vi "Autonomous Independent.vi"   [LabVIEW 2013]
doc: "This VI is called when autonomous begins, and will automatically be terminated when autonomous ends. You can carry out timed or sensor driven robot movement independently without needing to return to the caller."
uses:
  Robot Global Data.vi
  <vilib>/Rock Robotics/WPI/RobotDrive/WPI_RobotDriveGetSetRefNum.vi
panel:
  # "Be sure to right-click and choose Data Operations>>Make Current Value default if you want to save the array values with the VI"
types:
  T1 = enum16{"ToPos2", "ToPos1", "Fire", "Wait", "ESTOP", "Reset", "ToLowPower", "ToHighPower"}
  T2 = typedef "WPI_MotorControlDeviceRef.ctl" = cluster{"DeviceStatus":errorcluster, "Type":enum16{"PWM", "CAN"}, "PWM":cluster{"Digital Module":T3, "PWM Channel":T4, "DeadBand":T5}, "CAN":cluster{"Device Number":u8, "Control Mode":T6, "Semaphore":T7, "Max Vout":dbl}, "Invert":bool, "TransformRef":T8, "InvTransformRef":T8}
  T3 = typedef "FPGA_TypedefDigitalModule.ctl" = enum16{"Digital Module 1", "Digital Module 2"}
  T4 = typedef "FPGA_DIOPWMChannel.ctl" = enum8{"PWM 1", "PWM 2", "PWM 3", "PWM 4", "PWM 5", "PWM 6", "PWM 7", "PWM 8", "PWM 9", "PWM 10", "Invalid"}
  T5 = typedef "WPI_PWMDeadband.ctl" = cluster{"Name":string, "maxPositivePwm":i32, "minPositivePwm":i32, "centerPwm":i32, "maxNegativePwm":i32, "minNegativePwm":i32, "angularRange":u16}
  T6 = typedef "WPI_CANJaguar_ControlMode.ctl" = enum8{"Percent VBus", "Current", "Speed", "Position", "Voltage"}
  T7 = typedef "Semaphore RefNum" = refnum<k1>
  T8 = typedef "WPI_PWMTransform_ConPane.ctl" = refnum<vi>
  T9 = cluster{"UpLimit":bool, "Up2":bool, "Center":bool, "Down2":bool, "DownLimit":bool, "HighPowerLimit":bool, "EncoderRRate":dbl, "EncoderLRate":dbl, "ThumperE":dbl, "EncoderRDis":dbl, "EncoderLDis":dbl}
  T10 = typedef "WPI_RobotDriveDevRef.ctl" = cluster{"DevStatus":errorcluster, "Motors[]":T2[], "Square Inputs":bool, "Max Output":dbl, "Isochronous":bool}
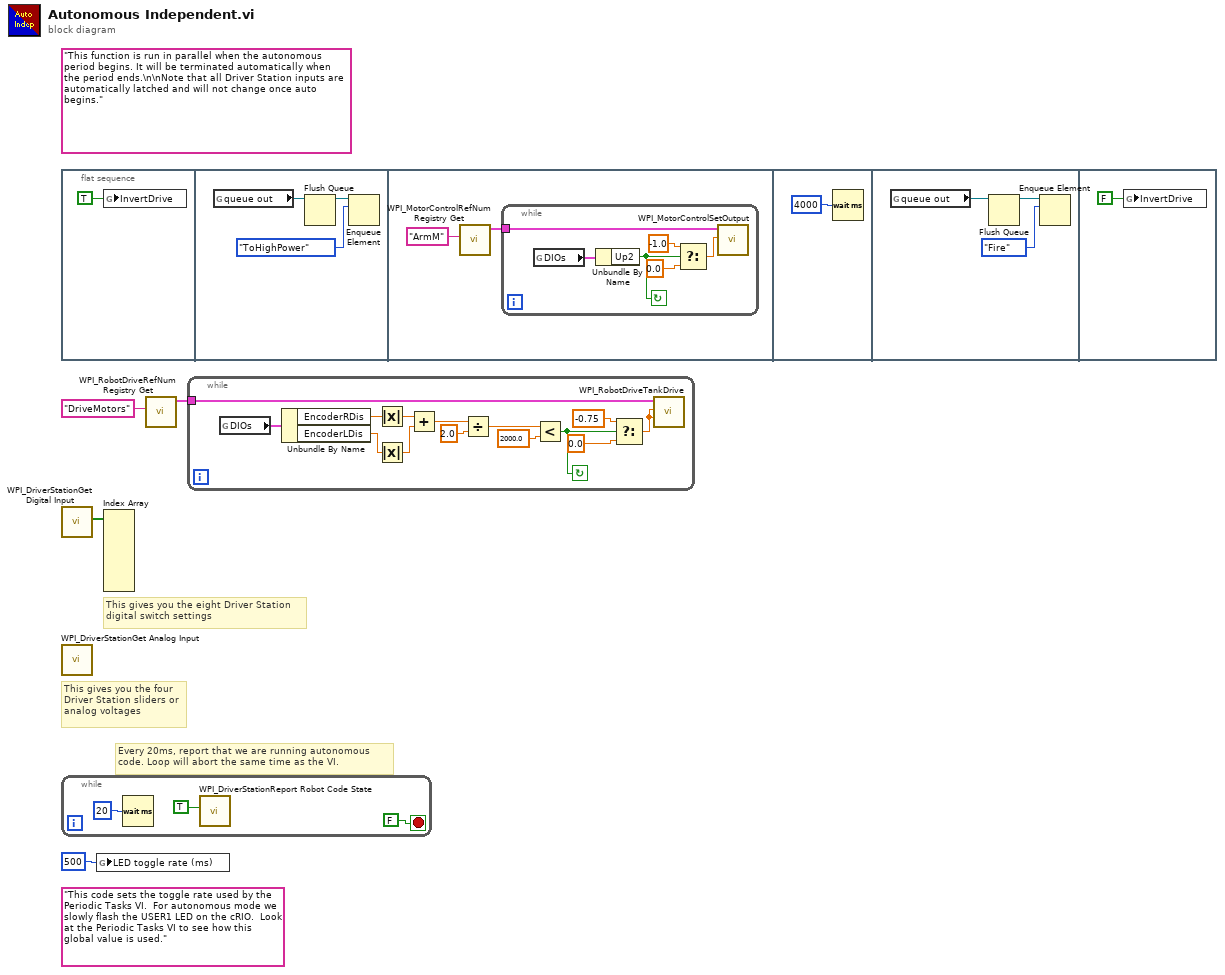
[diagram p0: block diagram]
diagram:
  (unwired) "This code sets the toggle rate used by the Periodic Tasks VI.  For autonomous mode we slowly flash the USER1 LED on the cRIO.  Look at the Periodic Tasks VI to see how this global value is used."
  (unwired) "This function is run in parallel when the autonomous period begins. It will be terminated automatically when the period ends.\n\nNote that all Driver Station inputs are automatically latched and will not change once auto begins."
  # "Every 20ms, report that we are running autonomous\ncode. Loop will abort the same time as the VI."
  # "This gives you the eight Driver Station\ndigital switch settings"
  # "This gives you the four\nDriver Station sliders or\nanalog voltages"
  n1 = flat-sequence {
    frame #0 {
      n2 = global write "Robot Global Data.vi" "InvertDrive"(TRUE) -> ()
    }
    frame #1 {
      n3 = global read "Robot Global Data.vi" "queue out"() -> (w6:refnum<queue>)
      n4 = Flush Queue(queue=w6) -> (queue out=w7:refnum<queue>)  [unwired: 1 in, 2 out]
      n5 = Enqueue Element(queue=w7, element=T1."ToHighPower") -> ()  [unwired: 2 in, 3 out]
    }
    frame #2 {
      n6 = call <vilib>:"WPI_MotorControlRefNum Registry Get.vi"("refnum name"="ArmM") -> ("MotorControlDevRef"=w9:T2)  [unwired: 9 in, 1 out]
      n7 = while {
        tunnel: w9 -> [w14]
        stop <- w12 continue-if-true
        n8 = global read "Robot Global Data.vi" "DIOs"() -> (w16:T9)
        n9 = Unbundle By Name(w16) -> ("Up2"=w12:bool)
        n10 = Select(t=-1.0, s=w12, f=0.0) -> (s? t:f=w15:dbl)
        n11 = call <vilib>:"WPI_MotorControlSetOutput.vi"("Output"=w15, "MotorControlDevRef"=w14) -> ()  [unwired: 7 in, 3 out]
      }
    }
    frame #3 {
      n12 = Wait (ms)(milliseconds to wait=u32 4000) -> ()  [unwired: 1 out]
    }
    frame #4 {
      n13 = global read "Robot Global Data.vi" "queue out"() -> (w20:refnum<queue>)
      n14 = Flush Queue(queue=w20) -> (queue out=w19:refnum<queue>)  [unwired: 1 in, 2 out]
      n15 = Enqueue Element(queue=w19, element=T1."Fire") -> ()  [unwired: 2 in, 3 out]
    }
    frame #5 {
      n16 = global write "Robot Global Data.vi" "InvertDrive"(FALSE) -> ()
    }
  }
  n17 = call <vilib>:"WPI_DriverStationGet Digital Input.vi"() -> ("Driver Station Digital Input (1-8)"=w4:bool[])  [unwired: 11 out]
  n18 = call <vilib>:"WPI_DriverStationGet Analog Input.vi"() -> ()  [unwired: 12 out]
  n19 = while {
    stop <- FALSE stop-if-true
    n20 = Wait (ms)(milliseconds to wait=u32 20) -> ()  [unwired: 1 out]
    n21 = call <vilib>:"WPI_DriverStationReport Robot Code State.vi"("Autonomous"=TRUE) -> ()  [unwired: 10 in, 1 out]
  }
  n22 = global write "Robot Global Data.vi" "LED toggle rate (ms)"(u32 500 ("LED ms toggle rate")) -> ()
  n23 = Index Array(array=w4) -> ()  [unwired: 8 in, 8 out]
  n24 = call <vilib>:"WPI_RobotDriveRefNum Registry Get.vi"("refnum name"="DriveMotors") -> ("RobotDriveDevRef"=w1:T10)  [unwired: 9 in, 1 out]
  n25 = while {
    tunnel: w1 -> [w26]
    stop <- w29 continue-if-true
    n26 = global read "Robot Global Data.vi" "DIOs"() -> (w38:T9)
    n27 = Unbundle By Name(w38) -> ("EncoderRDis"=w37:dbl, "EncoderLDis"=w36:dbl)
    n28 = Absolute Value(x=w37) -> (abs(x)=w34:dbl)
    n29 = Absolute Value(x=w36) -> (abs(x)=w35:dbl)
    n30 = Add(x=w34, y=w35) -> (x+y=w33:dbl)
    n31 = Divide(x=w33, y=2.0) -> (x/y=w31:dbl)
    n32 = Less?(x=w31, y=2000.0) -> (x < y?=w29:bool)
    n33 = Select(t=-0.75, s=w29, f=0.0) -> (s? t:f=w25:dbl)
    n34 = call <vilib>:"WPI_RobotDriveTankDrive.vi"("Right axis value"=w25, "Left axis value"=w25, "RobotDriveDevRef"=w26) -> ()  [unwired: 6 in, 3 out]
  }
